vi "Set Up GUI For Next Run.vi"(8 "error in (no error)":errorcluster, 11 "Tamer in":refnum<class "Tamer.lvclass">) -> (0 "error out":errorcluster, 3 "Tamer out":refnum<class "Tamer.lvclass">)   [LabVIEW 2020, in "CIRCUS_uServices.lvlib" / "Tamer.lvlib" / "Tamer.lvclass"]
uses:
  Tamer.lvclass
  Tamer.lvclass/Tamer.ctl
  Monkey Summary.ctl
  Link Chain GUI.ctl
  TALOS/TALOS_PPL.lvlibp/Father of all uServices/Father of all uServices/Father of all uServices.lvclass
  TALOS/TALOS_PPL.lvlibp
  Run Utilities/TypeDefs/Monkey Status.ctl
  Run Utilities/Run Utilities.lvlib
  C:/Users/marco/Documents/GitHub_Lab/CIRCUS/TALOS/TALOS_PPL.lvlibp/Father of all uServices/Father of all uServices/Father of all uServices.lvclass
  C:/Users/marco/Documents/GitHub_Lab/CIRCUS/TALOS/TALOS_PPL.lvlibp/Ancestor/Ancestor/Ancestor.lvclass
  C:/Users/marco/Documents/GitHub_Lab/CIRCUS/TALOS/Actor Framework.lvlibp/1abvi3w/vi.lib/ActorFramework/Actor/Actor.lvclass
  C:/Users/marco/Documents/GitHub_Lab/CIRCUS/CIRCUS uServices et al/Tamer/Tamer.lvclass
  Run Utilities/Schedule/Schedule.lvclass
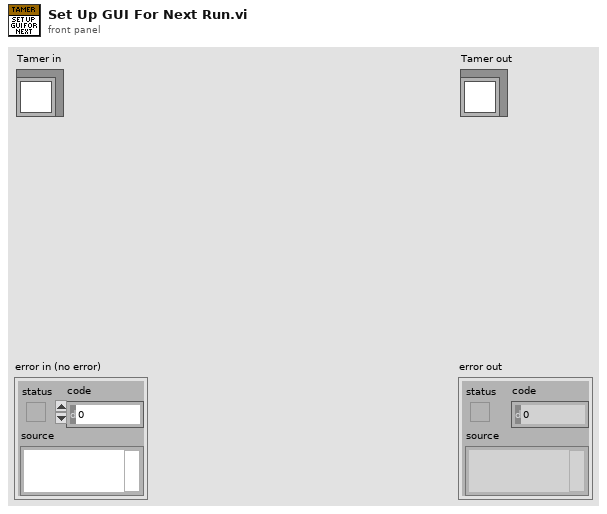
[diagram p1: front panel]
types:
  T1 = typedef "CIRCUS_uServices.lvlib/Tamer.lvlib/Tamer.lvclass/Monkey Summary.ctl" = cluster{"Color":u32, "Status":T2, "Continuous":bool, "Scripts left":u32, "Scripts skipped":u32, "ETA":string, "Current Action":string, "Report from previous RUNs":string, "Monkey ID":string, "With DAQ?":bool, "Linked?":T3, "Paused":bool}
  T2 = typedef "CIRCUS_uServices.lvlib/Run Utilities.lvlib/Monkey Status.ctl" = enum16{"Init", "Paused", "Ongoing", "Stopped", "Finished (no errors)", "Finished (with errors)"}
  T3 = typedef "CIRCUS_uServices.lvlib/Tamer.lvlib/Tamer.lvclass/Link Chain GUI.ctl" = bool
  T4 = typedef "CIRCUS_uServices.lvlib/Run Utilities.lvlib/Synchronize FPGA Cluster.ctl" = cluster{"Status":bool, "FPGA Name":string}
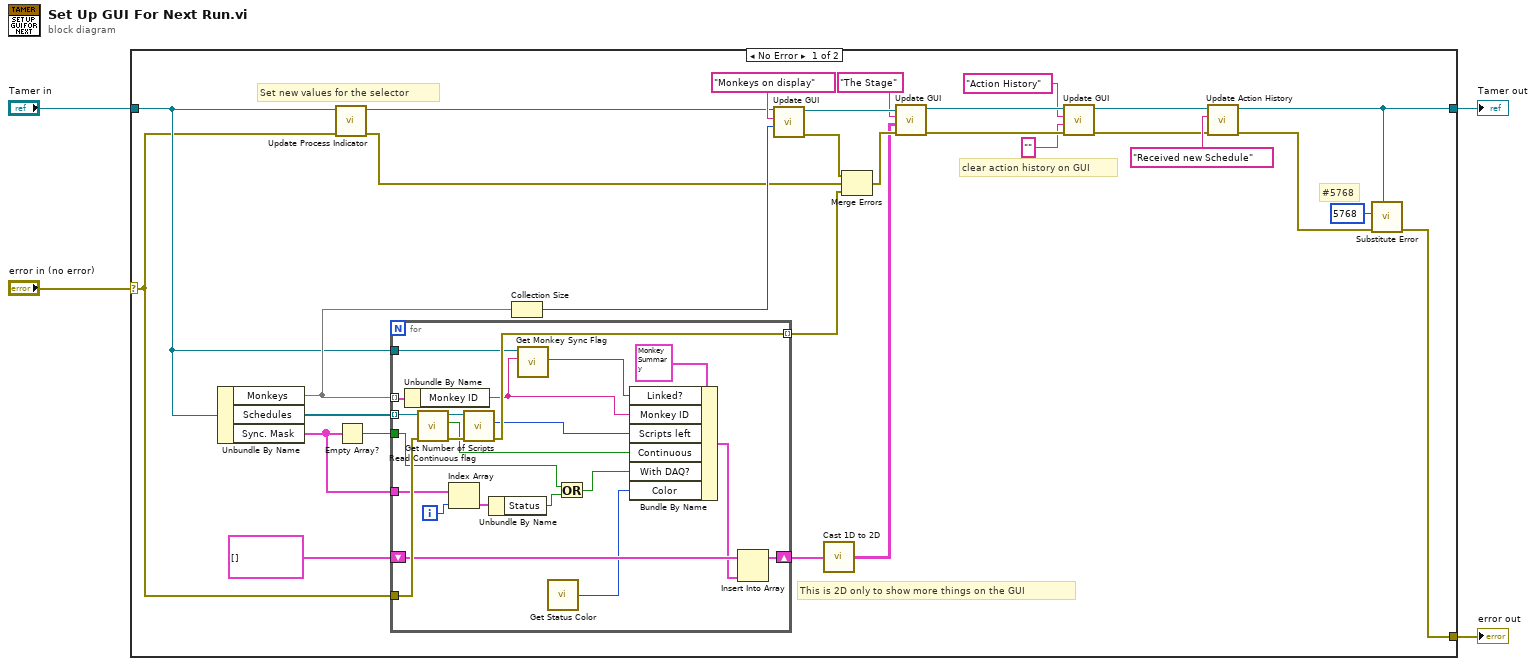
[diagram p0: block diagram]
diagram:
  n1 = case shown="No Error" "error in (no error)" {
    selector: "error in (no error)" -> [w10 w56]
    tunnel: [w27 w56] -> w3
    tunnel: [w25 w55] -> w1
    tunnel: "Tamer in" -> [w11 w55]
    frame No Error {
      # "clear action history on GUI"
      # "#5768"
      # "This is 2D only to show more things on the GUI"
      # "Set new values for the selector"
      n2 = Unbundle By Name(w11) -> ("Monkeys"=w17:map{string, string[]}, "Schedules"=w30:refnum<class "Schedule.lvclass">[], "Sync. Mask"=w14:T4[])
      n3 = call-dynamic "Update Process Indicator.vi"("error in (no error)"=w10, "Tamer in"=w11) -> ("error out"=w8:errorcluster, "Tamer out"=w9:refnum<class "Tamer.lvclass">)  [unwired: 8 in]
      n4 = Empty Array?(array=w14) -> (empty?=w28:bool)
      n5 = for {
        shift-right: [w49] -> w22
        shift-left: T1[] [] -> [w50]
        tunnel: w30 -> [w52] mode=indexing
        tunnel: w17 -> [w51] mode=indexing
        tunnel: w28 -> [w35]
        tunnel: w10 -> [w53]
        tunnel: [w54] -> w31 mode=indexing
        tunnel: w11 -> [w46]
        tunnel: w14 -> [w39]
        i -> [w38]
        n6 = Unbundle By Name(w51) -> ("Monkey ID"=w45:string)
        n7 = call-dynamic "Read Continuous flag.vi"("error in (no error)"=w53, "Schedule in"=w52) -> ("error out"=w42:errorcluster, "Continuous flag"=w40:bool, "Schedule out"=w43:refnum<class "Schedule.lvclass">)  [unwired: 7 in]
        n8 = Index Array(array=w39, index=w38) -> (element=w37:T4)
        n9 = call-dynamic "Get Number of Scripts.vi"("error in (no error)"=w42, "Schedule in"=w43) -> ("error out"=w54:errorcluster, "No. of Scripts"=w41:u32)  [unwired: 7 in, 1 out]
        n10 = Unbundle By Name(w37) -> ("Status"=w36:bool)
        n11 = call-dynamic "Get Monkey Sync Flag.vi"("Monkey ID"=w45, "Tamer in"=w46) -> ("Monkey Sync Flag"=w33:bool)  [unwired: 7 in, 2 out]
        n12 = call "Get Status Color.vi"() -> ("Color"=w44:u32)  [unwired: 1 in]
        n13 = Or(x=w35, y=w36) -> (x .or. y?=w34:bool)
        n14 = Bundle By Name(cluster=T1 {"Color"=16777225, "Status"=enum."Init", "Continuous"=FALSE, "Scripts left"=0, "Scripts skipped"=0, "ETA"="", "Current Action"="", "Report from previous RUNs"="", "Monkey ID"="", "With DAQ?"=FALSE, "Linked?"=FALSE, "Paused"=FALSE} ("Monkey Summary"), "Linked?"=w33, "Monkey ID"=w45, "Scripts left"=w41, "Continuous"=w40, "With DAQ?"=w34, "Color"=w44) -> (w47:T1)
        n15 = Insert Into Array(array=w50, new element=w47) -> (w49:T1[])  [unwired: 1 in]
      }
      n16 = Collection Size(1:w17) -> (0:w16:i32)
      n17 = call "Update GUI.vi"("Data"=w16, "GUI Item Name"="Monkeys on display", "uService Template in"=w9) -> ("error out"=w18:errorcluster, "uService Template out"=w19:refnum<class "Tamer.lvclass">)  [unwired: 7 in]
      n18 = call "Cast 1D to 2D.vi"("1D Monkeys"=w22) -> ("2D Monkeys"=w12:T1[][])
      n19 = Merge Errors(w18, w8, w31) -> (w21:errorcluster)
      n20 = call "Update GUI.vi"("error in (no error)"=w21, "Data"=w12, "GUI Item Name"="The Stage", "uService Template in"=w19) -> ("error out"=w15:errorcluster, "uService Template out"=w32:refnum<class "Tamer.lvclass">)  [unwired: 6 in]
      n21 = call "Update GUI.vi"("Data"="", "GUI Item Name"="Action History", "uService Template in"=w32) -> ("uService Template out"=w5:refnum<class "Tamer.lvclass">)  [unwired: 7 in, 1 out]
      n22 = call-dynamic "Update Action History.vi"("error in (no error)"=w15, "Action"="Received new Schedule", "Tamer in"=w5) -> ("error out"=w24:errorcluster, "Tamer out"=w25:refnum<class "Tamer.lvclass">)  [unwired: 7 in]
      n23 = call "Substitute Error.vi"("LabVIEW Object"=w25, "error in (no error)"=w24, "Error Code"=5768) -> ("error out"=w27:errorcluster)  [unwired: 8 in]
    }
    frame Error {
    }
  }
  "error out" <- w3
  "Tamer out" <- w1
